vi "Configure File.vi"(8 "Error In":errorcluster, 11 "Configuration":T1={"Delimiter"=",", "Enable Calendar Tree"=TRUE, "File Extension"="csv", "Maximum File Count"=5, "Maximum File Size"=15728640, "Prune All"=FALSE, "Root Folder"=path ""}) -> (0 "Error Out":errorcluster)   [LabVIEW 2025, in "LOGlib_LV2025.lvlib"]
doc: "All of the configurations for the default log file can be configured with this one VI instead of using VIs for each individual configuration. The individual configuration VIs are just wrappers around this VI."
uses:
  LOGlib_LV2025.lvlib
  Type Definitions/Configuration.ctl
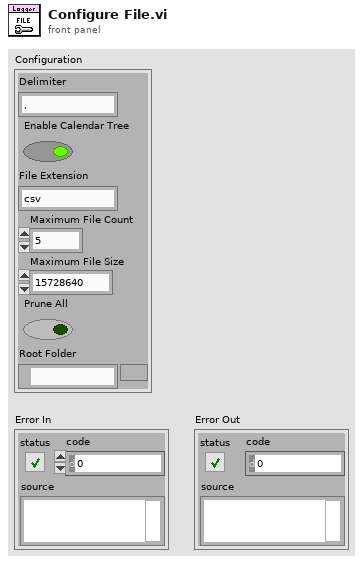
[diagram p1: front panel]
types:
  T1 = typedef "LOGlib_LV2025.lvlib/Configuration.ctl" = cluster{"Delimiter":string, "Enable Calendar Tree":bool, "File Extension":string, "Maximum File Count":i32, "Maximum File Size":i64, "Prune All":bool, "Root Folder":path}
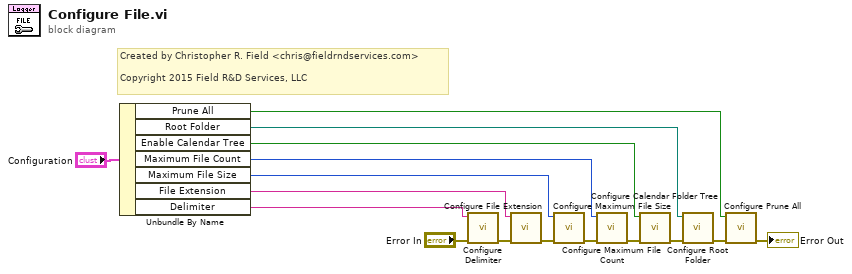
[diagram p0: block diagram]
diagram:
  # "Created by Christopher R. Field <chris@fieldrndservices.com>\n\nCopyright 2015 Field R&D Services, LLC"
  n1 = Unbundle By Name("Configuration") -> ("Prune All"=w4:bool, "Root Folder"=w12:path, "Enable Calendar Tree"=w13:bool, "Maximum File Count"=w7:i32, "Maximum File Size"=w8:i64, "File Extension"=w14:string, "Delimiter"=w1:string)
  n2 = call "Configure Delimiter.vi"("Error In"="Error In", "Delimiter"=w1) -> ("Error Out"=w2:errorcluster)  [unwired: 9 in]
  n3 = call "Configure File Extension.vi"("Error In"=w2, "File Extension"=w14) -> ("Error Out"=w9:errorcluster)  [unwired: 9 in]
  n4 = call "Configure Maximum File Size.vi"("Error In"=w9, "File Size"=w8) -> ("Error Out"=w10:errorcluster)  [unwired: 9 in]
  n5 = call "Configure Maximum File Count.vi"("Error In"=w10, "Maximum"=w7) -> ("Error Out"=w11:errorcluster)  [unwired: 9 in]
  n6 = call "Configure Calendar Folder Tree.vi"("Error In"=w11, "Enable"=w13) -> ("Error Out"=w15:errorcluster)  [unwired: 9 in]
  n7 = call "Configure Root Folder.vi"("Error In"=w15, "Root Folder"=w12) -> ("Error Out"=w6:errorcluster)  [unwired: 9 in]
  n8 = call "Configure Prune All.vi"("Error In"=w6, "Prune All"=w4) -> ("Error Out"=→"Error Out":errorcluster)  [unwired: 9 in]
